vi "SetValve.vi"(8 "Open/Close":bool, 11 "Valve":i32=32) -> ()   [LabVIEW 2011]
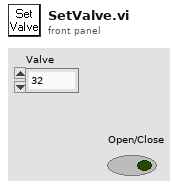
[diagram p1: front panel]
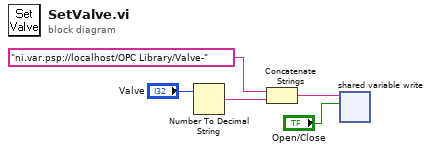
[diagram p0: block diagram]
diagram:
  n1 = Number To Decimal String(number="Valve") -> (decimal integer string=w5:string)  [unwired: 1 in]
  n2 = Concatenate Strings("ni.var.psp://localhost/OPC Library/Valve-", w5) -> (w2:string)
  n3 = shared-variable-write(w2, "Open/Close") -> ()  [unwired: 1 in, 2 out]
